vi "Enumerator go Previous.vi"(8 "error in (no error)":errorcluster, 11 "List in":refnum<class "DoubleLinkedList.lvclass">) -> (0 "error out":errorcluster, 3 "List out":refnum<class "DoubleLinkedList.lvclass">)   [LabVIEW 2010, in "DoubleLinkedList.lvclass"]
uses:
  DoubleLinkedList.lvclass
  DoubleLinkedList.lvclass/DoubleLinkedList.ctl
  ListNodeVirtual/ListNodeVirtual.lvclass
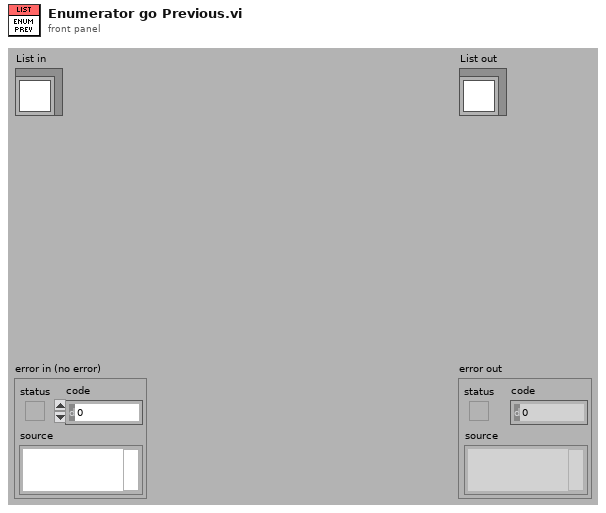
[diagram p1: front panel]
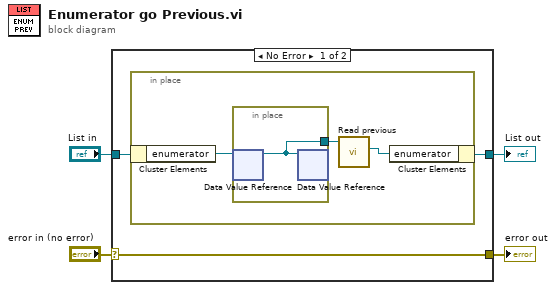
[diagram p0: block diagram]
diagram:
  n1 = case shown="No Error" "error in (no error)" {
    selector: "error in (no error)" -> [w7 w13]
    tunnel: [w7 w13] -> w3
    tunnel: [w5 w12] -> w1
    tunnel: "List in" -> [w6 w12]
    frame No Error {
      n2 = in-place {
        n3 = in-place-cluster #1(w6) -> ("enumerator"=w10:refnum<data-value>)
        n4 = in-place {
          in-place-border: [w11] -> w9
          n5 = in-place-dvr #2(w10) -> (w11:refnum<class "ListNodeVirtual.lvclass">)  [unwired: 1 out]
          n6 = in-place-dvr #2(w11) -> ()  [unwired: 2 out]
        }
        n7 = call-dynamic "Read previous.vi"("NodeType in"=w9) -> ("previous"=w8:refnum<data-value>)  [unwired: 8 in, 2 out]
        n8 = in-place-cluster #1("enumerator"=w8) -> (w5:refnum<class "DoubleLinkedList.lvclass">)
      }
    }
    frame Error {
    }
  }
  "error out" <- w3
  "List out" <- w1
